vi "Initialise.vi"(8 "error in (no error)":errorcluster, 11 "Node in":refnum<class "bt_Composite.lvclass">) -> (0 "error out":errorcluster, 3 "Node out":refnum<class "bt_Composite.lvclass">)   [LabVIEW 2021, in "BT.lvlib" / "bt_Composite.lvclass"]
uses:
  bt_Composite.lvclass
  bt_Composite.lvclass/bt_Composite.ctl
  abs_Node/bt_Node.lvclass
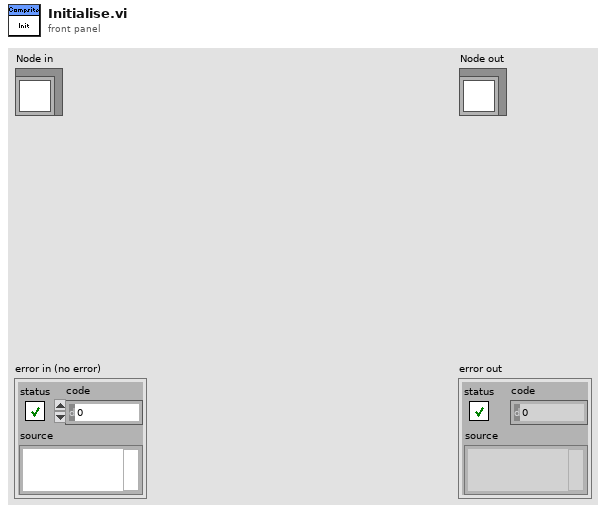
[diagram p1: front panel]
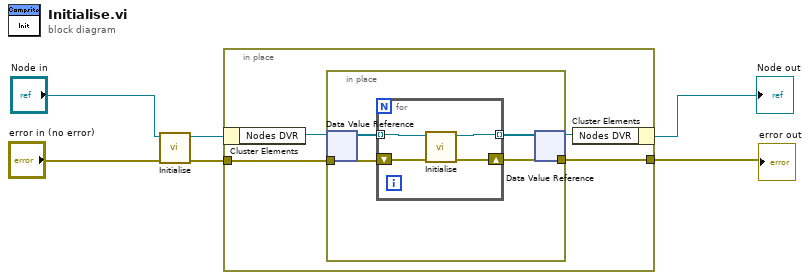
[diagram p0: block diagram]
diagram:
  n1 = call-parent "Initialise.vi"("error in (no error)"="error in (no error)", "Node in"="Node in") -> ("error out"=w1:errorcluster, "Node out"=w2:refnum<class "bt_Composite.lvclass">)  [unwired: 8 in]
  n2 = in-place {
    in-place-border: w1 -> [w8]
    in-place-border: [w7] -> w3
    n3 = in-place-cluster #1(w2) -> ("Nodes DVR"=w10:refnum<data-value>)
    n4 = in-place {
      in-place-border: w8 -> [w12]
      in-place-border: [w11] -> w7
      n5 = in-place-dvr #2(w10) -> (w14:refnum<class "bt_Node.lvclass">[])  [unwired: 1 out]
      n6 = for {
        tunnel: w14 -> [w18] mode=indexing
        tunnel: [w17] -> w13 mode=indexing
        shift-right: [w15] -> w11
        shift-left: w12 -> [w16]
        n7 = call-dynamic "Initialise.vi"("error in (no error)"=w16, "Node in"=w18) -> ("error out"=w15:errorcluster, "Node out"=w17:refnum<class "bt_Node.lvclass">)  [unwired: 8 in]
      }
      n8 = in-place-dvr #2(w13) -> (w9:refnum<data-value>)  [unwired: 1 out]
    }
    n9 = in-place-cluster #1("Nodes DVR"=w9) -> (→"Node out":refnum<class "bt_Composite.lvclass">)
  }
  "error out" <- w3
